vi "Get AI historian from PGserver.vi"(4 "time_min":timestamp, 6 "time_max":timestamp, 7 "k":dbl[](array[numeric])=[1.0, 1.0, 1.0, 1.0, 1.0, 1.0, 1.0, 1.0, 1.0, 1.0] min=0.01 max=1000.0 step=0.01, 8 "error in":errorcluster, 9 "ParamColumns":string[](array[string])=["EPBP1_XQ01", "EPBP2_XQ01", "EPBP3_XQ01"], 10 "ParamTable":string="EP_XQ.1802", 11 "conn":u32) -> (0 "error out":errorcluster, 3 "Out":cluster{timestamp[], dbl[]}[](array[cluster]))   [LabVIEW 2019, in "Inputs.lvlib"]
uses:
  Inputs.lvlib
  Database/PostgreSQL2LabVIEW/libpqlv/src/PQgetResult.vi
  Database/PostgreSQL2LabVIEW/libpqlv/src/PQclear.vi
  Database/PostgreSQL2LabVIEW/libpqUtility/src/PQfetchResultDataNotrans.vi
  Database/PostgreSQL2LabVIEW/libpqlv/src/PQresultErrorMessage.vi
  Database/PostgreSQL2LabVIEW/libpqlv/src/PQresultStatus.vi
  Database/PostgreSQL2LabVIEW/libpqlv/src/PQsendQuery.vi
  Database/PostgreSQL2LabVIEW/libpqlv/src/PQnfields.vi
  Database/PostgreSQL2LabVIEW/libpqlv/src/PQntuples.vi
  Database/PostgreSQL2LabVIEW/libpqlv/src/PQgetvalue.vi
  Database/PostgreSQL.lvlib
  Database/PostgreSQL2LabVIEW/libpqUtility/libpqutility.lvlib
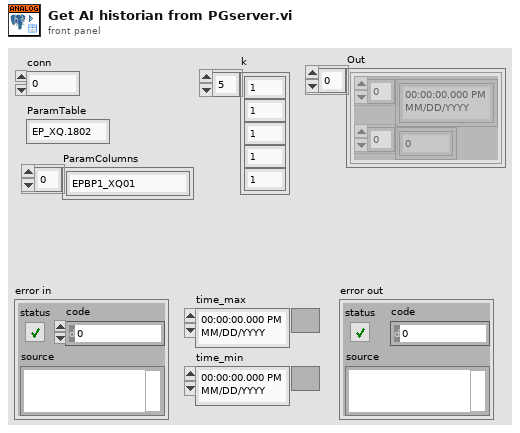
[diagram p1: front panel]
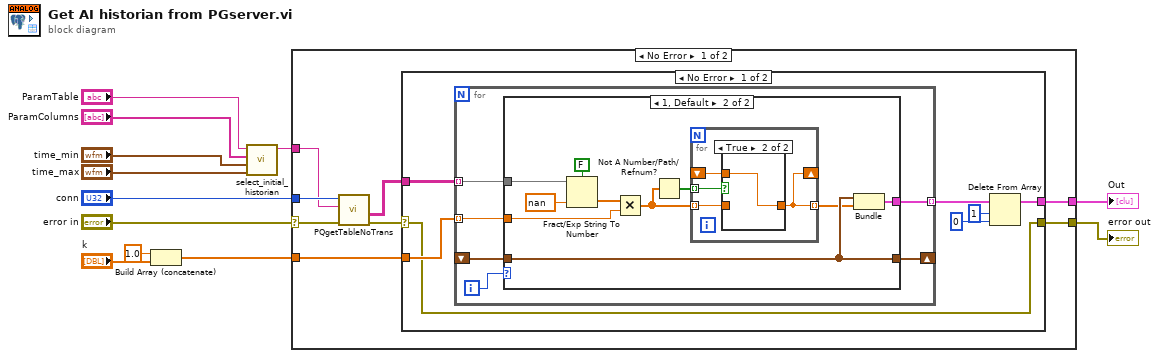
[diagram p0: block diagram]
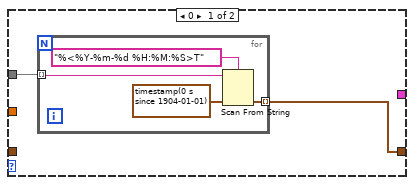
[diagram p2: hidden frame]
diagram:
  n1 = Build Array (concatenate)(1.0 ("element"), "k") -> (w6:dbl[])
  n2 = call "select_initial_historian.vi"("time_max"="time_max", "time_min"="time_min", "Column table"="ParamColumns", "table"="ParamTable") -> ("parameters"=w3:string)  [unwired: 7 in]
  n3 = case shown="No Error" "error in" {
    selector: "error in" -> [w18 w57]
    tunnel: "conn" -> [w19 _]
    tunnel: w3 -> [w17 _]
    tunnel: [w13 w57] -> w5
    tunnel: w6 -> [w20 _]
    tunnel: [w15 _] -> w9
    frame No Error {
      n4 = call "PQgetTableNoTrans.vi"("error in"=w18, "query"=w17, "conn"=w19) -> ("error out"=w14:errorcluster, "Data"=w16:string[][])  [unwired: 4 in, 3 out]
      n5 = case shown="No Error" w14 {
        selector: w14 -> [w21 w56]
        tunnel: w20 -> [w24 _]
        tunnel: w16 -> [w23 _]
        tunnel: [w22 _] -> w15
        tunnel: [w21 w56] -> w13
        frame No Error {
          n6 = for {
            tunnel: [w32] -> w27 mode=indexing
            tunnel: w23 -> [w30] mode=indexing
            tunnel: w24 -> [w31] mode=indexing
            shift-right: [w29] -> _
            shift-left: _ -> [w28]
            i -> [w33]
            n7 = case shown="1, Default" w33 {
              tunnel: [w34 w49] -> w29
              tunnel: w30 -> [w35 w46]
              tunnel: w28 -> [_ w49]
              tunnel: [_ w48] -> w32
              tunnel: w31 -> [_ w47]
              frame 0 {
                n8 = for {
                  tunnel: [w36] -> w34 mode=indexing
                  tunnel: w35 -> [w37] mode=indexing
                  n9 = Scan From String(format string="%<%Y-%m-%d %H:%M:%S>T" ("string"), input string=w37, default 1=timestamp(0 s since 1904-01-01) ("time stamp")) -> (output 1=w36:timestamp)  [unwired: 2 in, 3 out]
                }
              }
              frame 1, Default {
                n10 = Fract/Exp String To Number(use system decimal point (T)=FALSE, string=w46, default (0 dbl)=nan) -> (number=w42:dbl[])  [unwired: 1 in, 1 out]
                n11 = Multiply(x=w42, y=w47) -> (x*y=w41:dbl[])
                n12 = Not A Number/Path/Refnum?(number/path/refnum=w41) -> (NaN/Path/Refnum?=w40:bool[])
                n13 = for {
                  tunnel: [w51] -> w45 mode=indexing
                  tunnel: w41 -> [w53] mode=indexing
                  tunnel: w40 -> [w52] mode=indexing
                  shift-right: [w51] -> _
                  shift-left: _ -> [w50]
                  n14 = case shown="True" w52 {
                    tunnel: w53 -> [w54 _]
                    tunnel: [w54 w55] -> w51
                    tunnel: w50 -> [_ w55]
                    frame False {
                    }
                    frame True {
                    }
                  }
                }
                n15 = Bundle(w49, w45) -> (w48:cluster{timestamp[], dbl[]})  [unwired: 1 in]
              }
            }
          }
          n16 = Delete From Array(array=w27, length=1, index=0) -> (array with subset deleted=w22:cluster{timestamp[], dbl[]}[])  [unwired: 1 out]
        }
        frame Error {
        }
      }
    }
    frame Error {
    }
  }
  "Out" <- w9
  "error out" <- w5
